vi "igor define command_Cypher.vi"(11 "Command":string="td_ReadValue(\"difference%laser\")") -> (3 "History":string="%fprintf 0, \"%f\",td_ReadValue(\"difference%laser\")\r")   [LabVIEW 2016]
doc: "This VI will send commands to Igor."
panel:
  out "results":string="0.058594"
  out "error out":errorcluster
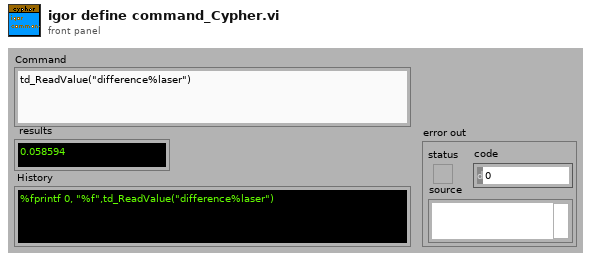
[diagram p1: front panel]
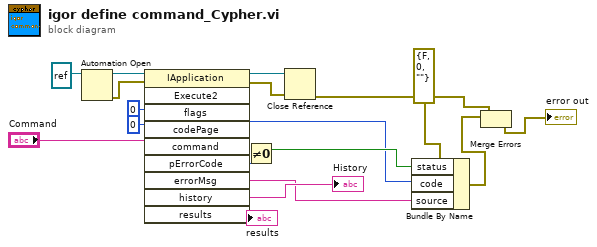
[diagram p0: block diagram]
diagram:
  n1 = Automation Open(Automation Refnum=refnum<k7> refnum ("IgorPro.IApplication")) -> (Automation Refnum=w17:refnum<k7>, error out=w16:errorcluster)  [unwired: 1 in, 2 out]
  n2 = invoke class="IApplication" method="Execute2"(reference=w17, error in=w16, "flags"=0, "codePage"=0, "command"="Command") -> (reference out=w15:refnum<k7>, error out=w14:errorcluster, "pErrorCode"=w5:i32, "errorMsg"=w4:string, "history"=→"History":string, "results"=→"results":string)  [unwired: 5 in, 4 out]
  n3 = Not Equal To 0?(x=w5) -> (x != 0?=w6:bool)
  n4 = Close Reference(reference=w15, error in (no error)=w14) -> (error out=w2:errorcluster)
  n5 = Bundle By Name(cluster=errorcluster {"status"=FALSE, "code"=0, "source"=""} ("error out 2"), "status"=w6, "code"=w5, "source"=w4) -> (w3:errorcluster)
  n6 = Merge Errors(w2, w3) -> (→"error out":errorcluster)
